vi "LWXPS_TCLScriptExecuteAndWait.vi"(0 "XPS Reference IN":refnum<k24>, 5 "TCL File Name":string, 7 "Task Name":string, 9 "Input Parameters List":string, 11 "LabVIEW error IN":errorcluster) -> (4 "XPS Reference OUT":refnum<k24>, 6 "Returned error code":i32, 8 "XPS Error String":string, 10 "Output parameters list":string[](array[string]), 15 "LabVIEW error OUT":errorcluster)   [LabVIEW 2014]
uses:
  D:/XPSQ8_LabView_Library/Development/Source/Dll/Newport.XPS.CommandInterface.dll
  Dll/Newport.XPS.CommandInterface.dll
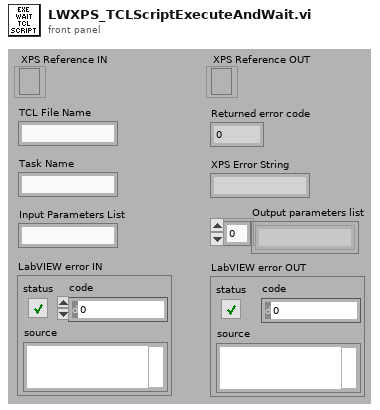
[diagram p1: front panel]
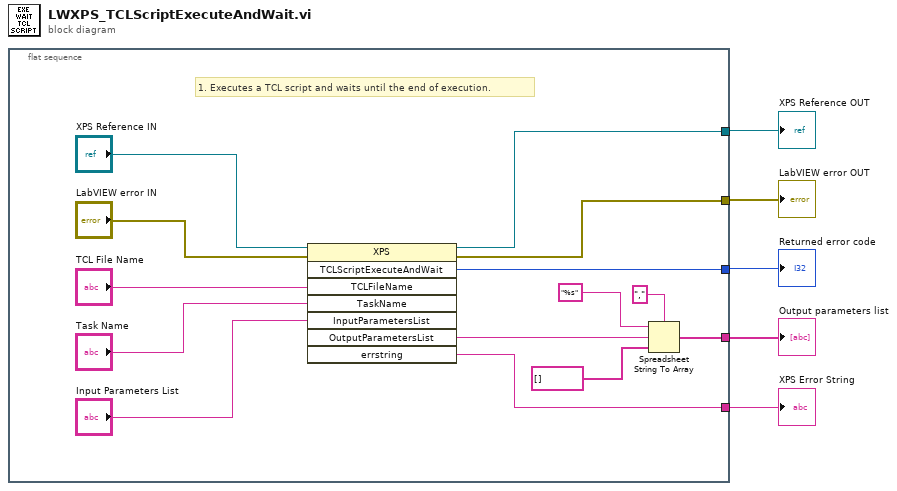
[diagram p0: block diagram]
diagram:
  n1 = flat-sequence {
    tunnel: [w15] -> w5
    tunnel: [w14] -> w4
    tunnel: [w16] -> w3
    tunnel: [w11] -> w2
    tunnel: [w6] -> w1
    frame #0 {
      # "1. Executes a TCL script and waits until the end of execution."
      n2 = invoke class="XPS" method="TCLScriptExecuteAndWait"(reference="XPS Reference IN", error in="LabVIEW error IN", "TCLFileName"="TCL File Name", "TaskName"="Task Name", "InputParametersList"="Input Parameters List") -> (reference out=w15:refnum<k24>, error out=w14:errorcluster, "TCLScriptExecuteAndWait"=w16:i32, "OutputParametersList"=w7:string, "errstring"=w11:string)  [unwired: 3 in, 3 out]
      n3 = Spreadsheet String To Array(delimiter (Tab)="," ("Delimiter (Tab)"), format string="%s" ("Format string"), spreadsheet string=w7, array type (2D Dbl)=string[] [] ("Type")) -> (array=w6:string[])
    }
  }
  "XPS Error String" <- w2
  "XPS Reference OUT" <- w5
  "LabVIEW error OUT" <- w4
  "Returned error code" <- w3
  "Output parameters list" <- w1
